vi "PH_Powermeter_BaseClass.PC get Energy.vi"(0 "i ref in":refnum<vi>, 2 "unscaled Energy [J]":dbl, 3 "Out of range?":bool, 5 "error in":errorcluster) -> (14 "i ref out":refnum<vi>, 19 "error out":errorcluster)   [LabVIEW 2014, in "PH_Powermeter_BaseClass.lvlib"]
doc: "This VI writes wanted Settings to the Device and checks the result."
uses:
  PH_Powermeter_BaseClass.lvlib
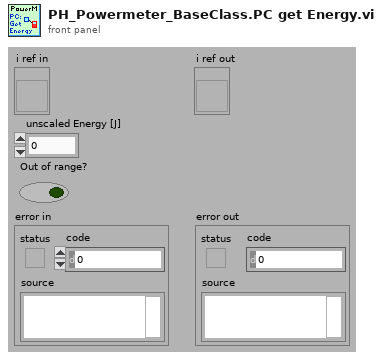
[diagram p1: front panel]
types:
  T1 = typedef "PH_Powermeter_BaseClass.lvlib/PH_Powermeter_BaseClass.i attribute.ctl" = cluster{"GUI References":T2, "Connection":T3, "Head Attributes":T5, "VISA resource":refnum<visa-resource-name>, "Energy":T6, "Service ID Energy":i32, "Wanted Settings":T7, "Current Settings":T7}
  T2 = typedef "PH_Powermeter_BaseClass.lvlib/PH_Powermeter_BaseClass.GUI Refs.ctl" = cluster{"Head Attributes":refnum<vi>, "Energy":refnum<vi>, "Connection":refnum<vi>, "VISA Resource":refnum<vi>, "Energy evolution":refnum<vi>, "Scaling Factor":refnum<vi>, "Range":refnum<vi>, "Wavelength":refnum<vi>, "Trigger Level":refnum<vi>, "Wanted Settings":refnum<vi>, "Current Settings":refnum<vi>}
  T3 = typedef "PH_Powermeter_BaseClass.lvlib/PH_Powermeter_BaseClass.Connection.ctl" = cluster{"failed checks":i8, "Timeout":bool, "Data read":string, "Failure":bool, "Error":bool, "State":T4}
  T4 = typedef "PH_Powermeter_BaseClass.lvlib/PH_Powermeter_BaseClass.State.ctl" = enum32{"off", "operating", "opened", "checked", "connected", "Sets to change", "running"}
  T5 = typedef "PH_Powermeter_BaseClass.lvlib/PH_Powermeter_BaseClass.Head Attributes.ctl" = cluster{"Instrument Type":string, "Head Version":string, "Head Name":string, "Serial Number":string, "Firmware":string, "Sensor Type":string, "MinimumRange":u32, "Maximum Range":u32, "Min Wavelength":i32, "Max Wavelength":i32}
  T6 = typedef "PH_Powermeter_BaseClass.lvlib/PH_Powermeter_BaseClass.Energy.ctl" = cluster{"current Value":dbl, "unscaled":dbl, "Scaling Factor":dbl}
  T7 = typedef "PH_Powermeter_BaseClass.lvlib/PH_gentec_BaseClass.Head Settings.ctl" = cluster{"Trigger Level":dbl, "Wavelength":u32, "Range":u32}
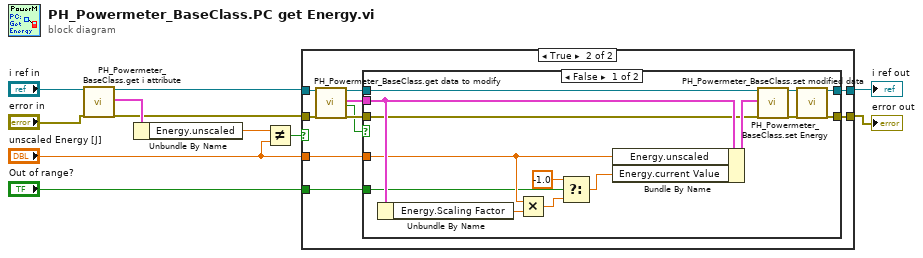
[diagram p0: block diagram]
diagram:
  n1 = call "PH_Powermeter_BaseClass.get i attribute.vi"("i ref in"="i ref in", "error in (no error)"="error in") -> ("i ref out"=w5:refnum<vi>, "i attribute"=w8:T1, "error out"=w7:errorcluster)  [unwired: 15 in]
  n2 = Unbundle By Name(w8) -> ("Energy.unscaled"=w9:dbl)
  n3 = Not Equal?(x=w9, y="unscaled Energy [J]") -> (x != y?=w3:bool)
  n4 = case shown="True" w3 {
    tunnel: [w12 w23] -> w11
    tunnel: [w13 w22] -> w10
    tunnel: w7 -> [w12 w17]
    tunnel: w5 -> [w13 w16]
    tunnel: "unscaled Energy [J]" -> [_ w15]
    tunnel: "Out of range?" -> [_ w14]
    frame False {
    }
    frame True {
      n5 = call "PH_Powermeter_BaseClass.get data to modify.vi"("i ref in"=w16, "error in (no error)"=w17) -> ("i ref out"=w20:refnum<vi>, "i attribute"=w19:T1, "timed out"=w18:bool, "error out"=w21:errorcluster)  [unwired: 14 in]
      n6 = case shown="False" w18 {
        tunnel: w15 -> [w31 _]
        tunnel: [w28 w39] -> w22
        tunnel: [w30 w38] -> w23
        tunnel: w21 -> [w32 w38]
        tunnel: w20 -> [w37 w39]
        tunnel: w19 -> [w34 _]
        tunnel: w14 -> [w27 _]
        frame False {
          n7 = Unbundle By Name(w34) -> ("Energy.Scaling Factor"=w33:dbl)
          n8 = Multiply(x=w31, y=w33) -> (x*y=w24:dbl)
          n9 = Select(t=-1.0, s=w27, f=w24) -> (s? t:f=w26:dbl)
          n10 = Bundle By Name(cluster=w34, "Energy.unscaled"=w31, "Energy.current Value"=w26) -> (w35:T1)
          n11 = call "PH_Powermeter_BaseClass.set modified data.vi"("i ref in"=w37, "i attribute"=w35, "error in (no error)"=w32) -> ("i ref out"=w29:refnum<vi>, "error out"=w36:errorcluster)  [unwired: 15 in]
          n12 = call "PH_Powermeter_BaseClass.set Energy.vi"("VI in"=w29, "error in (no error)"=w36) -> ("VI out"=w28:refnum<vi>, "error out"=w30:errorcluster)  [unwired: 16 in]
        }
        frame True {
        }
      }
    }
  }
  "error out" <- w11
  "i ref out" <- w10
